vi "Elevator Loop.vi"(0 "Elevator Enc":T1, 1 "Elevator":T4={"DeviceStatus"={"status"=FALSE, "code"=0, "source"=""}, "Type"=enum."PWM", "PWM"={"Digital Module"=enum."Digital Module 1", "PWM Channel"=enum."Invalid", "DeadBand"={"Name"="", "maxPositivePwm"=0, "minPositivePwm"=0, "centerPwm"=0, "maxNegativePwm"=0, "minNegativePwm"=0, "angularRange"=0}}, "CAN"={"Device Number"=0, "Control Mode"=enum."Percent VBus", "Semaphore"=refnum, "Max Vout"=12.0}, "Invert"=FALSE, "TransformRef"=refnum, "InvTransformRef"=refnum}, 2 "Personality":string, 3 "Elev Stable Tol (sec)":dbl, 4 "Auto Pitch":bool=TRUE) -> ()   [LabVIEW 2012]
uses:
  <vilib>/Rock Robotics/WPI/MotorControl/WPI_MotorControlDeviceRef.ctl
  <vilib>/Rock Robotics/SystemInterfaces/Typedef/FPGA_TypedefDigitalModule.ctl
  <vilib>/Rock Robotics/SystemInterfaces/DIO/FPGA_DIOPWMChannel.ctl
  <vilib>/Rock Robotics/WPI/PWM/WPI_PWMDeadband.ctl
  <vilib>/Rock Robotics/WPI/CAN/Jaguar/SubVIs/WPI_CANJaguar_ControlMode.ctl
  <vilib>/Rock Robotics/WPI/PWM/WPI_PWMTransform_ConPane.ctl
  <vilib>/Rock Robotics/WPI/AnalogChannel/WPI_AnalogChannelDevRef.ctl
  <vilib>/Rock Robotics/SystemInterfaces/Typedef/FPGA_TypedefAnalogModule.ctl
  <vilib>/Rock Robotics/SystemInterfaces/AI/FPGA_AIChannel.ctl
  <vilib>/addons/control/pid/pid.llb/PID (DBL).vi
  <vilib>/addons/control/pid/NI_PID_pid.lvlib
panel:
  in  "max climb pitch":dbl=30.0
  out "Pitch Voltage":dbl(slide) scale=0.0..5.0
  in  "Elevator Motor Test":dbl(knob) scale=-0.2..0.2
  out "Voltage":dbl
  in  "Speed limit":dbl=0.6
  out "Pitch (deg)":dbl
  in  "Prop":dbl(knob)=0.10043892521573479 scale=0.0..0.2
  in  "Int":dbl(knob)=0.0047421871896915985 scale=0.0..0.02
  in  "Der":dbl(knob) scale=0.0..0.01
  in  "Test ?":bool
  out "Pitch":cluster{"ElevatorControl":dbl, dbl}(graph)
  in  "Amplify":dbl(knob)=6.139372973419566 scale=0.0..10.0
  in  "SineBypass":bool
  in  "Feeder Station Load Angle":dbl=29.0
  out "Elevator Stable 2":bool
  in  "Elev Tol":dbl=0.9
  in  "Sense at Lo":dbl=3.57
  in  "Sense at Hi":dbl=3.0
  in  "Lo Mech":dbl=15.7
  in  "Hi Mech":dbl=29.7
  in  "Hi Mech B":dbl=29.7
  in  "Lo Mech B":dbl=13.5
  in  "Sense at Hi B":dbl=2.9
  in  "Sense at Lo B":dbl=3.65
  in  "Asym+":dbl
  in  "Asym-":dbl=0.08
  in  "Asym+ B":dbl
  in  "Asym- B":dbl=0.04
  in  "Elevator Angle during climb":dbl=20.0
  in  "Pelican":dbl=0.3
  in  "PBot Offset":dbl
  out "At Hi":bool
  out "At Lo":bool
  in  "Lo Limit":dbl=17.0
  in  "Hi Limit":dbl=34.5
  in  "Near Limit (deg)":dbl
  in  "Motor Cuttout":dbl
  out "Motor is Cut Out":bool
  out "Motor Command":dbl=0.04
  out "Motor Output":dbl(knob) scale=-0.5..0.5
  # "Easy Cal Bot A"
  # "A: 3.58\nB: 3.34"
  # "A: 15.1\nB: 13.3"
  # "A: 40.3\nB: 42.9"
  # "A: 2.61\nB: 1.88"
  # "Easy Cal Bot B"
  # "37 deg at Palm"
  # "Elevator Up"
  # "Elevator Down"
  # "Min pwr = -0.11"
  # "Min pwr = 0.03"
  # "Bot A"
  # "Bot B"
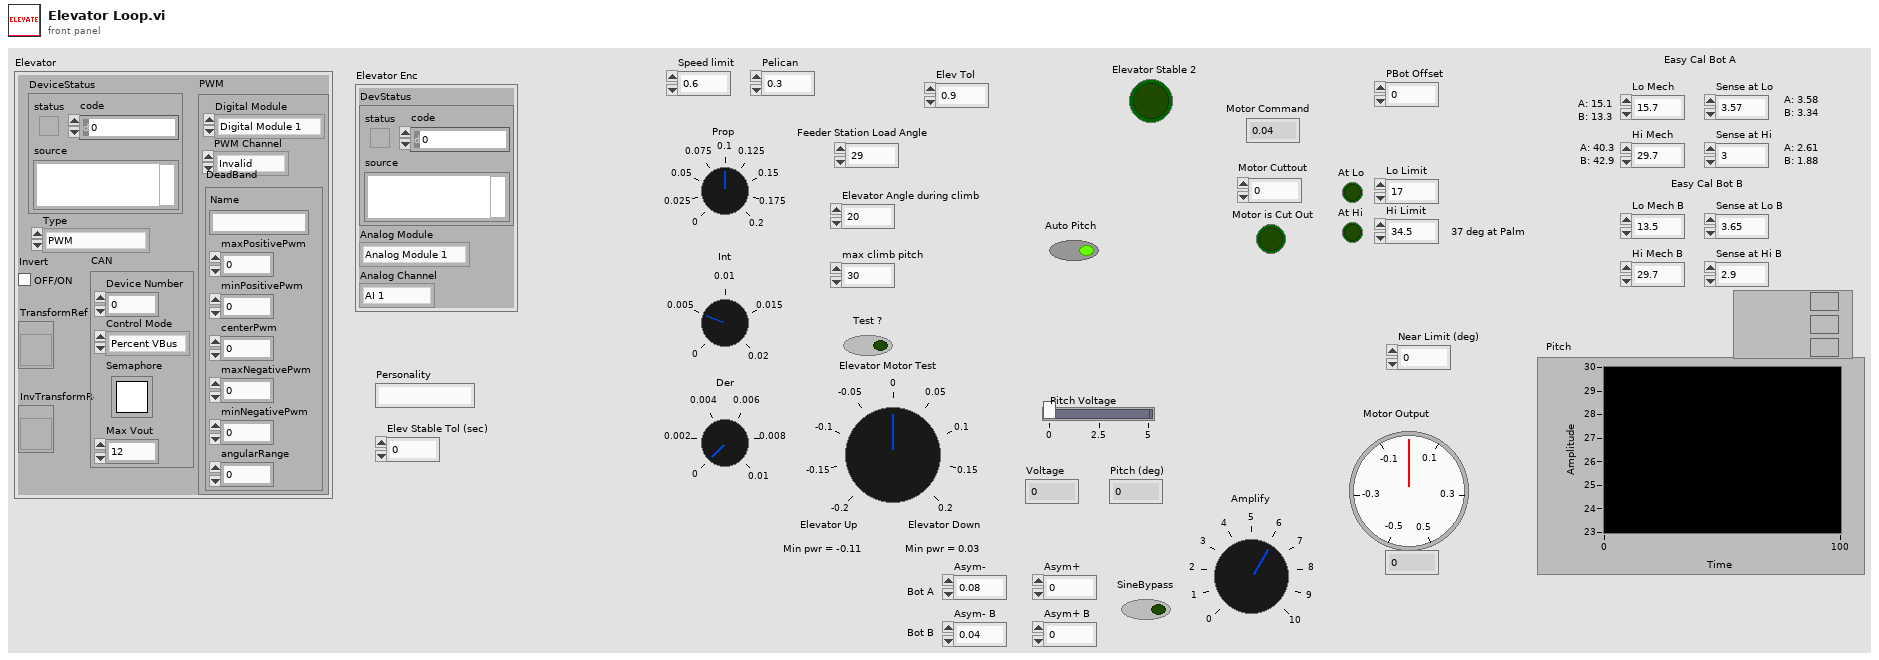
[diagram p1: front panel]
types:
  T1 = typedef "WPI_AnalogChannelDevRef.ctl" = cluster{"DevStatus":errorcluster, "Analog Module":T2, "Analog Channel":T3}
  T2 = typedef "FPGA_TypedefAnalogModule.ctl" = enum16{"Analog Module 1", "Analog Module 2"}
  T3 = typedef "FPGA_AIChannel.ctl" = enum8{"AI 1", "AI 2", "AI 3", "AI 4", "AI 5", "AI 6", "AI 7", "AI 8", "Invalid"}
  T4 = typedef "WPI_MotorControlDeviceRef.ctl" = cluster{"DeviceStatus":errorcluster, "Type":enum16{"PWM", "CAN"}, "PWM":cluster{"Digital Module":T5, "PWM Channel":T6, "DeadBand":T7}, "CAN":cluster{"Device Number":u8, "Control Mode":T8, "Semaphore":T9, "Max Vout":dbl}, "Invert":bool, "TransformRef":T10, "InvTransformRef":T10}
  T5 = typedef "FPGA_TypedefDigitalModule.ctl" = enum16{"Digital Module 1", "Digital Module 2"}
  T6 = typedef "FPGA_DIOPWMChannel.ctl" = enum8{"PWM 1", "PWM 2", "PWM 3", "PWM 4", "PWM 5", "PWM 6", "PWM 7", "PWM 8", "PWM 9", "PWM 10", "Invalid"}
  T7 = typedef "WPI_PWMDeadband.ctl" = cluster{"Name":string, "maxPositivePwm":i32, "minPositivePwm":i32, "centerPwm":i32, "maxNegativePwm":i32, "minNegativePwm":i32, "angularRange":u16}
  T8 = typedef "WPI_CANJaguar_ControlMode.ctl" = enum8{"Percent VBus", "Current", "Speed", "Position", "Voltage"}
  T9 = typedef "Semaphore RefNum" = refnum<k1>
  T10 = typedef "WPI_PWMTransform_ConPane.ctl" = refnum<vi>
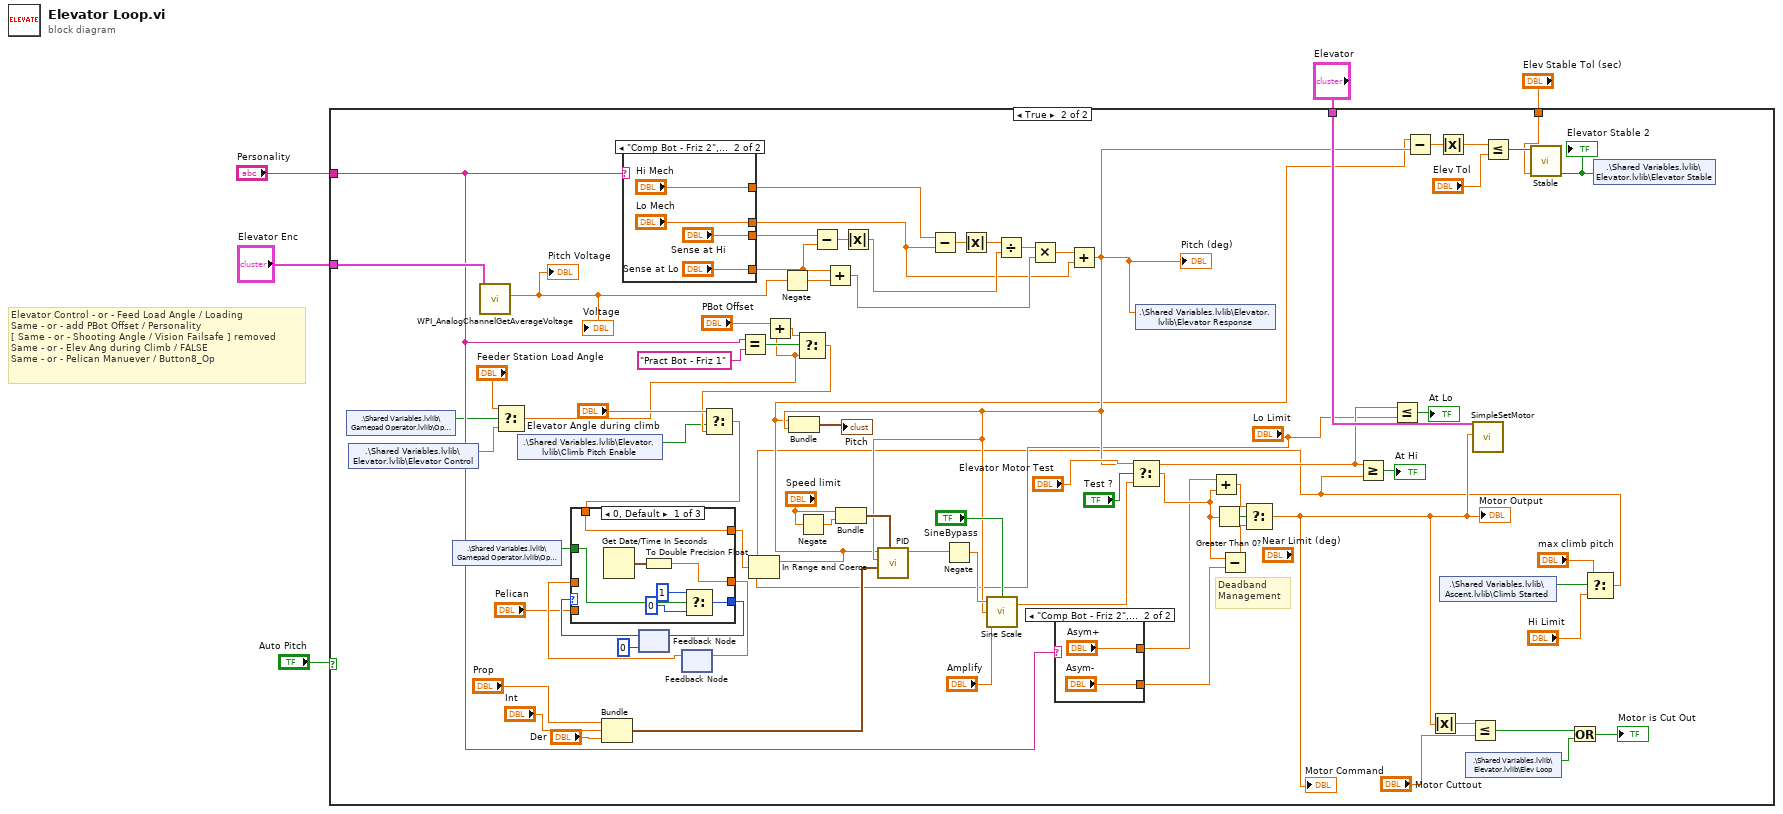
[diagram p0: block diagram]
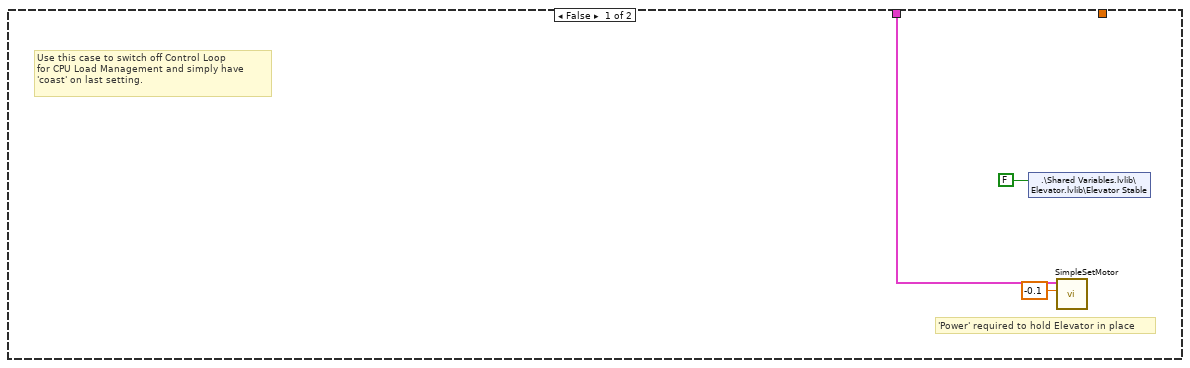
[diagram p2: hidden frame]
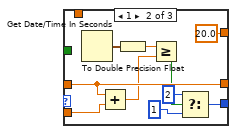
[diagram p3: hidden frame]
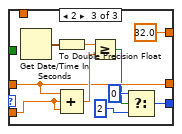
[diagram p4: hidden frame]
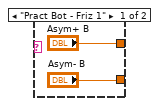
[diagram p5: hidden frame]
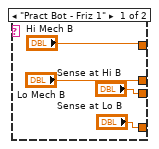
[diagram p6: hidden frame]
diagram:
  # "Elevator Control - or - Feed Load Angle / Loading\nSame - or - add PBot Offset / Personality\n[ Same - or - Shooting Angle / Vision Failsafe ] removed\nSame - or - Elev Ang during Climb / FALSE\nSame - or - Pelican Manuever / Button8_Op"
  n1 = case shown="True" "Auto Pitch" {
    tunnel: "Elevator" -> [w8 w86]
    tunnel: "Elevator Enc" -> [_ w85]
    tunnel: "Elev Stable Tol (sec)" -> [_ w54]
    tunnel: "Personality" -> [_ w42]
    frame False {
      # "'Power' required to hold Elevator in place"
      # "Use this case to switch off Control Loop\nfor CPU Load Management and simply have\n'coast' on last setting."
      n2 = shared-variable ".\\Shared Variables.lvlib\\Elevator.lvlib\\Elevator Stable"(FALSE ("Signal Input")) -> ()  [unwired: 1 in, 1 out]
      n3 = call "SimpleSetMotor.vi"("Output"=-0.1, "MotorControlDevRef"=w8) -> ()  [unwired: 8 in, 2 out]
    }
    frame True {
      # "Deadband\nManagement"
      n4 = shared-variable ".\\Shared Variables.lvlib\\Gamepad Operator.lvlib\\Op Button 4"() -> (w31:bool)  [unwired: 1 in, 1 out]
      n5 = shared-variable ".\\Shared Variables.lvlib\\Elevator.lvlib\\Elevator Control"() -> (w29:dbl)  [unwired: 1 in, 1 out]
      n6 = shared-variable ".\\Shared Variables.lvlib\\Gamepad Operator.lvlib\\Op Button 8"() -> (w30:bool)  [unwired: 1 in, 1 out]
      n7 = call <vilib>:"WPI_AnalogChannelGetAverageVoltage.vi"("AIDeviceRef"=w85) -> ("Voltage"=w14:dbl)  [unwired: 8 in, 2 out]
      "Pitch Voltage" <- w14
      "Voltage" <- w14
      n8 = Select(t="Feeder Station Load Angle", s=w31, f=w29) -> (s? t:f=w32:dbl)
      n9 = shared-variable ".\\Shared Variables.lvlib\\Elevator.lvlib\\Climb Pitch Enable"() -> (w13:bool)  [unwired: 1 in, 1 out]
      n10 = Bundle("Prop"="Prop", "Int"="Int", "Der"="Der") -> (w81:cluster{"Prop":dbl, "Int":dbl, "Der":dbl})  [unwired: 1 out]
      n11 = case shown="\"Comp Bot - Friz 2\", Default" w42 {
        tunnel: ["Sense at Lo B" "Sense at Lo"] -> w66
        tunnel: ["Sense at Hi B" "Sense at Hi"] -> w65
        tunnel: ["Hi Mech B" "Hi Mech"] -> w50
        tunnel: ["Lo Mech B" "Lo Mech"] -> w49
        frame "Pract Bot - Friz 1" {
        }
        frame "Comp Bot - Friz 2", Default {
        }
      }
      n12 = feedback #1(0 ("t")) -> (w39:i32)
      n13 = feedback #2() -> (w36:dbl)  [unwired: 1 in]
      n14 = Equal?(x=w42, y="Pract Bot - Friz 1") -> (x = y?=w45:bool)
      n15 = Add(x="PBot Offset", y=w32) -> (x+y=w46:dbl)
      n16 = Negate(x=w14) -> (-x=w64:dbl)
      n17 = Select(t=w46, s=w45, f=w32) -> (s? t:f=w28:dbl)
      n18 = Select(t="Elevator Angle during climb", s=w13, f=w28) -> (s? t:f=w38:dbl)
      n19 = case shown="0, Default" w39 {
        tunnel: [w93 w98 w108] -> w40
        tunnel: w38 -> [w90 _ _]
        tunnel: [w90 20.0 32.0 ("ElevatorControl")] -> w17
        tunnel: w30 -> [w91 _ _]
        tunnel: [w87 w101 w106] -> w37
        tunnel: w36 -> [_ w101 w106]
        tunnel: "Pelican" -> [_ w94 w104]
        frame 0, Default {
          n20 = Get Date/Time In Seconds() -> (seconds since 1Jan1904=w88:timestamp)
          n21 = To Double Precision Float(number=w88) -> (double precision float=w87:dbl)
          n22 = Select(t=1, s=w91, f=0) -> (s? t:f=w93:i32)
        }
        frame 1 {
          n23 = Get Date/Time In Seconds() -> (seconds since 1Jan1904=w102:timestamp)
          n24 = Add(x=w101, y=w94) -> (x+y=w99:dbl)
          n25 = To Double Precision Float(number=w102) -> (double precision float=w100:dbl)
          n26 = Greater Or Equal?(x=w100, y=w99) -> (x >= y?=w96:bool)
          n27 = Select(t=2, s=w96, f=1) -> (s? t:f=w98:i32)
        }
        frame 2 {
          n28 = Get Date/Time In Seconds() -> (seconds since 1Jan1904=w112:timestamp)
          n29 = To Double Precision Float(number=w112) -> (double precision float=w111:dbl)
          n30 = Compound Arithmetic op=ADD(w106, w104, w104) -> (w107:dbl)
          n31 = Greater Or Equal?(x=w111, y=w107) -> (x >= y?=w105:bool)
          n32 = Select(t=0, s=w105, f=2) -> (s? t:f=w108:i32)
        }
      }
      n33 = feedback-in #1(w40) -> ()
      n34 = feedback-in #2(w37) -> ()
      n35 = Negate(x="Speed limit") -> (-x=w84:dbl)
      n36 = Subtract(x=w65, y=w66) -> (x-y=w67:dbl)
      n37 = Add(x=w66, y=w64) -> (x+y=w72:dbl)
      n38 = Bundle("Speed limit"="Speed limit", w84) -> (w82:cluster{"Speed limit":dbl, dbl})  [unwired: 1 out]
      n39 = Absolute Value(x=w67) -> (abs(x)=w70:dbl)
      n40 = Subtract(x=w50, y=w49) -> (x-y=w68:dbl)
      n41 = Absolute Value(x=w68) -> (abs(x)=w69:dbl)
      n42 = Divide(x=w69, y=w70) -> (x/y=w71:dbl)
      n43 = Multiply(x=w71, y=w72) -> (x*y=w73:dbl)
      n44 = case shown="\"Comp Bot - Friz 2\", Default" w42 {
        tunnel: ["Asym+ B" "Asym+"] -> w48
        tunnel: ["Asym- B" "Asym-"] -> w47
        frame "Pract Bot - Friz 1" {
        }
        frame "Comp Bot - Friz 2", Default {
        }
      }
      n45 = Add(x=w73, y=w49) -> (x+y=w18:dbl)
      "Pitch (deg)" <- w18
      n46 = shared-variable ".\\Shared Variables.lvlib\\Elevator.lvlib\\Elevator Response"(w18) -> ()  [unwired: 1 in, 1 out]
      n47 = Less Or Equal?(x=w18, y="Lo Limit") -> (x <= y?=→"At Lo":bool)
      n48 = shared-variable ".\\Shared Variables.lvlib\\Ascent.lvlib\\Climb Started"() -> (w12:bool)  [unwired: 1 in, 1 out]
      n49 = shared-variable ".\\Shared Variables.lvlib\\Elevator.lvlib\\Elev Loop"() -> (w20:bool)  [unwired: 1 in, 1 out]
      n50 = Select(t="max climb pitch", s=w12, f="Hi Limit") -> (s? t:f=w9:dbl)
      n51 = In Range and Coerce(upper limit=w9, x=w17, lower limit="Lo Limit") -> (coerced(x)=w16:dbl)  [unwired: 1 out]
      n52 = Bundle("Hi Limit"=w16, w18) -> (→"Pitch":cluster{"Hi Limit":dbl, dbl})  [unwired: 1 out]
      n53 = call-poly <vilib>:"PID.vi"("output range"=w82, "PID gains"=w81, "process variable"=w18, "setpoint"=w16) -> ("output"=w75:dbl)  [unwired: 2 in, 5 out]
      n54 = Negate(x=w75) -> (-x=w62:dbl)
      n55 = call "Sine Scale.vi"("bypass"="SineBypass", "Amplify"="Amplify", "Sensor"=w18, "Input"=w62) -> ("Output"=w52:dbl)  [unwired: 1 in]
      n56 = Select(t="Elevator Motor Test", s="Test ?", f=w52) -> (s? t:f=w58:dbl)
      n57 = Add(x=w48, y=w58) -> (x+y=w59:dbl)
      n58 = Greater Than 0?(x=w58) -> (x > 0?=w61:bool)
      n59 = Subtract(x=w58, y=w47) -> (x-y=w60:dbl)
      n60 = Select(t=w59, s=w61, f=w60) -> (s? t:f=w19:dbl)
      "Motor Command" <- w19
      "Motor Output" <- w19
      n61 = Greater Or Equal?(x=w18, y=w9) -> (x >= y?=→"At Hi":bool)
      n62 = Subtract(x=w16, y=w18) -> (x-y=w57:dbl)
      n63 = Absolute Value(x=w19) -> (abs(x)=w23:dbl)
      n64 = Absolute Value(x=w57) -> (abs(x)=w56:dbl)
      n65 = Less Or Equal?(x=w23, y="Motor Cuttout") -> (x <= y?=w24:bool)
      n66 = call "SimpleSetMotor.vi"("Output"=w19, "MotorControlDevRef"=w86) -> ()  [unwired: 8 in, 2 out]
      n67 = Less Or Equal?(x=w56, y="Elev Tol") -> (x <= y?=w55:bool)
      n68 = call "Stable.vi"("Eval Period (sec)"=w54, "Signal Input"=w55) -> ("Stable"=w27:bool)  [unwired: 9 in]
      "Elevator Stable 2" <- w27
      n69 = Or(x=w24, y=w20) -> (x .or. y?=→"Motor is Cut Out":bool)
      n70 = shared-variable ".\\Shared Variables.lvlib\\Elevator.lvlib\\Elevator Stable"(w27) -> ()  [unwired: 1 in, 1 out]
    }
  }
